vi "SingleCounter-trig_start_stop_update.vi"(10 "Duration_s":dbl) -> (0 "error out":errorcluster, 1 "triggers_task":refnum<k21>, 2 "Waveform Graph":u32[](graph), 3 "APD_task":refnum<k21>)   [LabVIEW 2018]
uses:
  GLOBAL_VAR.vi
  <vilib>/DAQmx/create/channels.llb/DAQmx Create Channel (CI-Count Edges).vi
  <vilib>/DAQmx/configure/timing.llb/DAQmx Timing (Sample Clock).vi
  <resource>/objmgr/daqmx.rc
  <vilib>/DAQmx/read.llb/DAQmx Read (Counter 1D U32 1Chan NSamp).vi
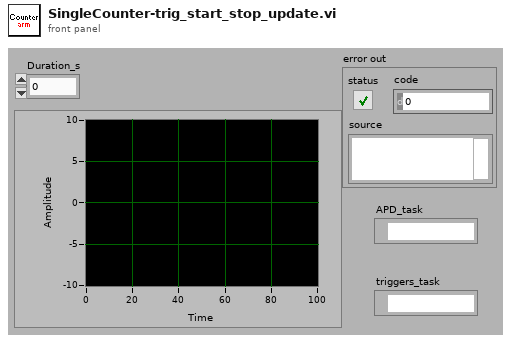
[diagram p1: front panel]
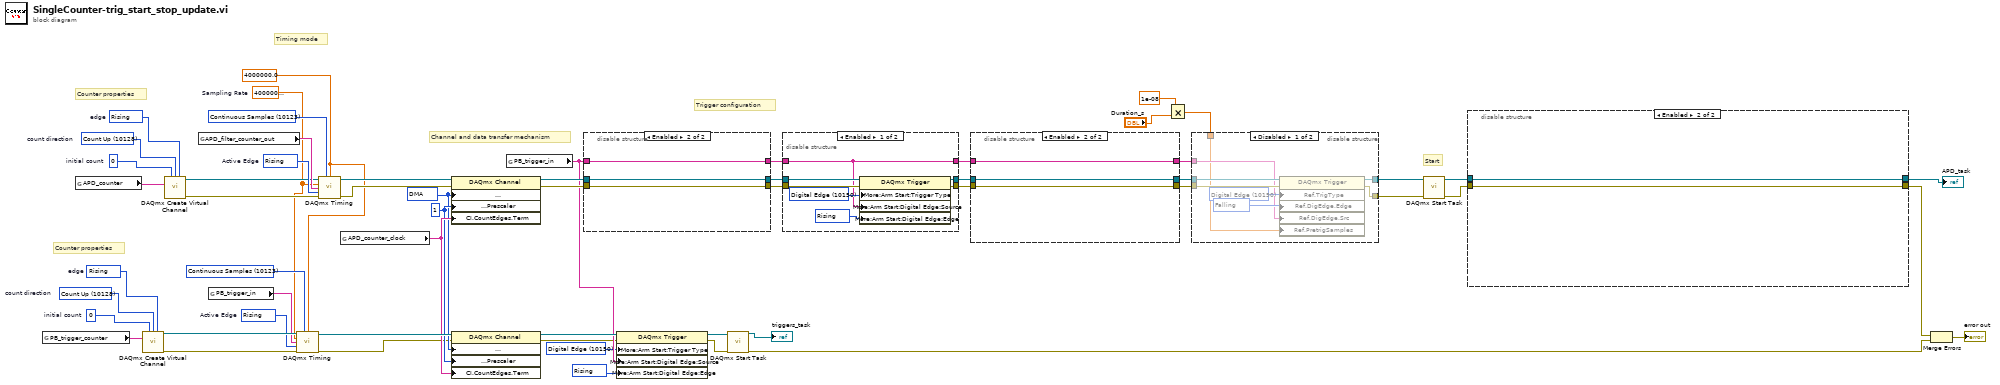
[diagram p0: block diagram]
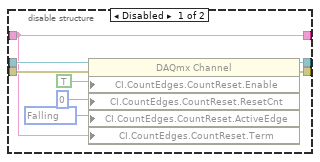
[diagram p4: hidden frame]
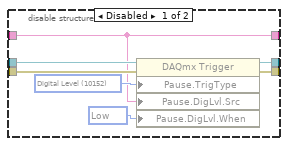
[diagram p5: hidden frame]
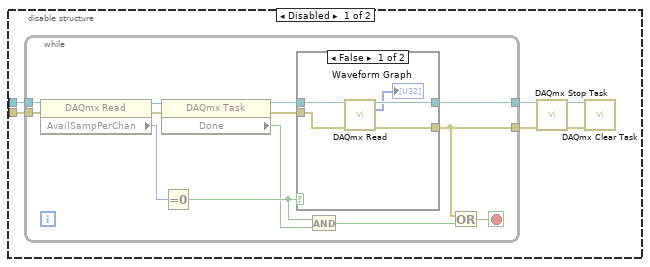
[diagram p6: hidden frame]
diagram:
  w4 = 4000000.0
  w14 = 10150 items=["Digital Edge"=10150, "None"=10230] ("Trigger Type")
  w13 = 10280 items=["Rising"=10280, "Falling"=10171] ("Trigger Edge")
  w25 = 10280 items=["Rising"=10280, "Falling"=10171]  # Active Edge
  w23 = 10123 items=["Finite Samples"=10178, "Continuous Samples"=10123, "Hardware Timed Single Point"=12522] ("Sample Mode")
  w29 = 10128 items=["Count Up"=10128, "Count Down"=10124, "Externally Controlled"=10326]  # count direction
  w30 = 10280 items=["Rising"=10280, "Falling"=10171]  # edge
  w28 = u32 0  # initial count
  w22 = 40000000.0  # Sampling Rate
  w18 = u32 1 ("CI.Prescaler")
  w57 = 10280 items=["Rising"=10280, "Falling"=10171]  # Active Edge
  w55 = 10128 items=["Count Up"=10128, "Count Down"=10124, "Externally Controlled"=10326]  # count direction
  w56 = 10280 items=["Rising"=10280, "Falling"=10171]  # edge
  w54 = u32 0  # initial count
  w17 = 10054 items=["DMA"=10054, "Interrupts"=10204, "Programmed I/O"=10264] ("CI.DataXferMech")
  w53 = 10123 items=["Finite Samples"=10178, "Continuous Samples"=10123, "Hardware Timed Single Point"=12522] ("Sample Mode")
  # "Counter properties"
  # "Trigger configuration"
  # "Counter properties"
  # "Channel and data transfer mechanism"
  # "Timing mode"
  # "Start"
  n1 = global read "GLOBAL_VAR.vi" "PB_trigger_counter"() -> (w27:tag)
  n2 = global read "GLOBAL_VAR.vi" "APD_counter"() -> (w50:tag)
  n3 = call-poly <vilib>:"DAQmx Create Virtual Channel.vi"("initial count"=w28, "count direction"=w29, "edge"=w30, "counter"=w27) -> ("task out"=w26:refnum<k21>, "error out"=w21:errorcluster)  [unwired: 10 in]
  n4 = call-poly <vilib>:"DAQmx Create Virtual Channel.vi"("initial count"=w54, "count direction"=w55, "edge"=w56, "counter"=w50) -> ("task out"=w48:refnum<k21>, "error out"=w47:errorcluster)  [unwired: 10 in]
  n5 = global read "GLOBAL_VAR.vi" "APD_filter_counter_out"() -> (w49:tag)
  n6 = global read "GLOBAL_VAR.vi" "PB_trigger_in"() -> (w24:tag)
  n7 = call-poly <vilib>:"DAQmx Timing.vi"("task/channels in"=w26, "sample mode"=w23, "samples per channel"=w4, "rate"=w22, "source"=w24, "active edge"=w25, "error in"=w21) -> ("task out"=w20:refnum<k21>, "error out"=w9:errorcluster)  [unwired: 7 in]
  n8 = call-poly <vilib>:"DAQmx Timing.vi"("task/channels in"=w48, "sample mode"=w53, "samples per channel"=w4, "rate"=w22, "source"=w49, "active edge"=w57, "error in"=w47) -> ("task out"=w45:refnum<k21>, "error out"=w46:errorcluster)  [unwired: 7 in]
  n9 = global read "GLOBAL_VAR.vi" "APD_counter_clock"() -> (w19:tag)
  n10 = property class="DAQmx Channel"(reference=w45, error in=w46, "Counter Input:General Properties:More:Advanced:Data Transfer and Memory:Data Transfer Mechanism"=w17, "Counter Input:General Properties:More:Advanced:Prescaler"=w18, "CI.CountEdges.Term"=w19) -> (reference out=w41:refnum<k21>, error out=w40:errorcluster)
  n11 = property class="DAQmx Channel"(reference=w20, error in=w9, "Counter Input:General Properties:More:Advanced:Data Transfer and Memory:Data Transfer Mechanism"=w17, "Counter Input:General Properties:More:Advanced:Prescaler"=w18, "CI.CountEdges.Term"=w19) -> (reference out=w16:refnum<k21>, error out=w10:errorcluster)
  n12 = global read "GLOBAL_VAR.vi" "PB_trigger_in"() -> (w15:tag)
  n13 = disable-structure shown="Enabled" {
    disable-tunnel: w41 -> [w64 w67]
    disable-tunnel: w40 -> [w63 w66]
    disable-tunnel: [w60 w67] -> w39
    disable-tunnel: [w59 w66] -> w38
    disable-tunnel: [w58 w65] -> w31
    disable-tunnel: w15 -> [w58 w65]
    frame Disabled {
      w61 = 10214 items=["High"=10192, "Low"=10214] ("Pause.DigLvl.When")
      w62 = 10152 items=["Analog Level"=10101, "Analog Window"=10103, "Digital Level"=10152, "Digital Pattern"=10398, "None"=10230] ("Pause.TrigType")
      n14 = property class="DAQmx Trigger"(reference=w64, error in=w63, "Pause.TrigType"=w62, "Pause.DigLvl.Src"=w58, "Pause.DigLvl.When"=w61) -> (reference out=w60:refnum<k21>, error out=w59:errorcluster)
    }
    frame Enabled {
    }
  }
  n15 = property class="DAQmx Trigger"(reference=w16, error in=w10, "More:Arm Start:Trigger Type"=w14, "More:Arm Start:Digital Edge:Source"=w15, "More:Arm Start:Digital Edge:Edge"=w13) -> (reference out=w12:refnum<k21>, error out=w11:errorcluster)
  n16 = call <vilib>:"DAQmx Start Task.vi"("task/channels in"=w12, "error in"=w11) -> ("task out"=→"triggers_task":refnum<k21>, "error out"=w5:errorcluster)  [unwired: 12 in]
  n17 = disable-structure shown="Enabled" {
    disable-tunnel: [w74 w77] -> w43
    disable-tunnel: [w73 w76] -> w42
    disable-tunnel: w39 -> [w72 w77]
    disable-tunnel: w38 -> [w71 w76]
    disable-tunnel: w31 -> [w68 w75]
    disable-tunnel: [w68 w75] -> w32
    frame Enabled {
      w70 = 10150 items=["Digital Edge"=10150, "None"=10230] ("Trigger Type")
      w69 = 10280 items=["Rising"=10280, "Falling"=10171] ("Trigger Edge")
      n18 = property class="DAQmx Trigger"(reference=w72, error in=w71, "More:Arm Start:Trigger Type"=w70, "More:Arm Start:Digital Edge:Source"=w68, "More:Arm Start:Digital Edge:Edge"=w69) -> (reference out=w74:refnum<k21>, error out=w73:errorcluster)
    }
    frame Disabled {
    }
  }
  n19 = disable-structure shown="Enabled" {
    disable-tunnel: w43 -> [w85 w88]
    disable-tunnel: w42 -> [w84 w87]
    disable-tunnel: [w83 w88] -> w37
    disable-tunnel: [w82 w87] -> w36
    disable-tunnel: w32 -> [w78 w86]
    disable-tunnel: [w78 w86] -> w33
    frame Disabled {
      w79 = 10171 items=["Rising"=10280, "Falling"=10171] ("CI.CountEdges.CountReset.ActiveEdge")
      n20 = property class="DAQmx Channel"(reference=w85, error in=w84, "CI.CountEdges.CountReset.Enable"=TRUE, "CI.CountEdges.CountReset.ResetCnt"=u32 0, "CI.CountEdges.CountReset.ActiveEdge"=w79, "CI.CountEdges.CountReset.Term"=w78) -> (reference out=w83:refnum<k21>, error out=w82:errorcluster)
    }
    frame Enabled {
    }
  }
  n21 = Multiply(x=1e-08, y="Duration_s") -> (x*y=w1:dbl)
  n22 = disable-structure shown="Disabled" {
    disable-tunnel: w37 -> [w96 w98]
    disable-tunnel: w36 -> [w95 w97]
    disable-tunnel: [w92 w98] -> w35
    disable-tunnel: [w89 w97] -> w34
    disable-tunnel: w33 -> [w91 _]
    disable-tunnel: w1 -> [w90 _]
    frame Disabled {
      w93 = 10171 items=["Rising"=10280, "Falling"=10171] ("Ref.DigEdge.Edge")
      w94 = 10150 items=["Analog Edge"=10099, "Digital Edge"=10150, "Digital Pattern"=10398, "Analog Window"=10103, "None"=10230] ("Ref.TrigType")
      n23 = property class="DAQmx Trigger"(reference=w96, error in=w95, "Ref.TrigType"=w94, "Ref.DigEdge.Edge"=w93, "Ref.DigEdge.Src"=w91, "Ref.PretrigSamples"=w90) -> (reference out=w92:refnum<k21>, error out=w89:errorcluster)
    }
    frame Enabled {
    }
  }
  n24 = call <vilib>:"DAQmx Start Task.vi"("task/channels in"=w35, "error in"=w34) -> ("task out"=w51:refnum<k21>, "error out"=w52:errorcluster)  [unwired: 12 in]
  n25 = disable-structure shown="Enabled" {
    disable-tunnel: w52 -> [w104 w125]
    disable-tunnel: w51 -> [w103 w126]
    disable-tunnel: [_ w126] -> w44
    disable-tunnel: [_ w125] -> w7
    frame Disabled {
      n26 = while {
        tunnel: w104 -> [w115]
        tunnel: w103 -> [w114]
        tunnel: [w110] -> w100
        tunnel: [w108] -> w99
        stop <- w109 stop-if-true
        n27 = property class="DAQmx Read"(reference=w114, error in=w115) -> (reference out=w117:refnum<k21>, error out=w116:errorcluster, "AvailSampPerChan"=w113:u32)
        n28 = property class="DAQmx Task"(reference=w117, error in=w116) -> (reference out=w112:refnum<k21>, error out=w111:errorcluster, "Done"=w105:bool)
        n29 = Equal To 0?(x=w113) -> (x = 0?=w106:bool)
        n30 = case shown="False" w106 {
          tunnel: w112 -> [w122 w124]
          tunnel: w111 -> [w121 w123]
          tunnel: [w120 w124] -> w110
          tunnel: [w119 w123] -> w108
          frame False {
            n31 = call-poly <vilib>:"DAQmx Read.vi"("task/channels in"=w122, "error in"=w121) -> ("task out"=w120:refnum<k21>, "data"=→"Waveform Graph":u32[], "error out"=w119:errorcluster)  [unwired: 11 in]
          }
          frame True {
          }
        }
        n32 = And(x=w106, y=w105) -> (x .and. y?=w107:bool)
        n33 = Or(x=w108, y=w107) -> (x .or. y?=w109:bool)
      }
      n34 = call <vilib>:"DAQmx Stop Task.vi"("task/channels in"=w100, "error in"=w99) -> ("task out"=w102:refnum<k21>, "error out"=w101:errorcluster)  [unwired: 12 in]
      n35 = call <vilib>:"DAQmx Clear Task.vi"("task in"=w102, "error in"=w101) -> ()  [unwired: 13 in, 1 out]
    }
    frame Enabled {
    }
  }
  "APD_task" <- w44
  n36 = Merge Errors(w7, w5) -> (→"error out":errorcluster)
